vi "Fetch Multi Eval Meas List Segment SEM Margin Area Results.vi"(6 "Offset Frequency (Negative)":i32(ring) items=["Negative", "Positive"], 7 "Segment (1)":T2=1, 8 "error in (no error)":errorcluster, 9 "Result Type (Current)":i32(ring) items=["Current"=0, "Average"=1, "Minimum"=5], 10 "Instance (1)":T3=1, 11 "VISA resource name":refnum<visa-resource-name>) -> (0 "error out":errorcluster, 1 "SEM Offset Results":cluster{"Margin X":dbl, "Margin Y":dbl}[](array[cluster]) {"Margin Y" format="%^.3e"; "Margin X" format="%^.3e"}, 2 "Reliability Results":T1, 3 "VISA resource name out":refnum<visa-resource-name>, 4 "Statistic Expired":i32, 5 "Out Of Tolerance":dbl format="%^.3e")   [LabVIEW 2020, in "Rohde&Schwarz CMXP NR FR2 Measurement.lvlib"]
doc: "Returns spectrum emission mask margin results for segment <no> in list mode.\n\nAttributes:\nRSCMXPNRFR2M_ATTR_FETCH_MULTI_EVAL_MEASUREMENT_LIST_SEGMENT_SEM_NEGATIVE_CURRENT_RESULTS\nRSCMXPNRFR2M_ATTR_FETCH_MULTI_EVAL_MEASUREMENT_LIST_SEGMENT_SEM_NEGATIVE_AVERAGE_RESULTS\nRSCMXPNRFR2M_ATTR_FETCH_MULTI_EVAL_MEASUREMENT_LIST_SEGMENT_SEM_NEGATIVE_MINIMUM_RESULTS\nRSCMXPNRFR2M_ATTR_FETCH_MULTI_EVAL_MEASUREMENT_LIST_SEGMENT_SEM_POSITIVE_CURRENT_RESULTS\nRSCMXPNRFR2M_ATTR_FETCH_MULTI_EVAL_MEASUREMENT_LIST_SEGMENT_SEM_POSITIVE_AVERAGE_RESULTS\nRSCMXPNRFR2M_ATTR_FETCH_MULTI_EVAL_MEASUREMENT_LIST_SEGMENT_SEM_POSITIVE_MINIMUM_RESULTS\n\nRemote-control commands:\nFETCh:NRMMw:MEAS<i>:MEValuation:LIST:SEGMent<no>:SEMask:MARGin:CURRent:NEGativ?\nFETCh:NRMMw:MEAS<i>:MEValuation:LIST:SEGMent<no>:SEMask:MARGin:AVERage:NEGativ?\nFETCh:NRMMw:MEAS<i>:MEValuation:LIST:SEGMent<no>:SEMask:MARGin:MINimum:NEGativ?\nFETCh:NRMMw:MEAS<i>:MEValuation:LIST:SEGMent<no>:SEMask:MARGin:CURRent:POSitiv?\nFETCh:NRMMw:MEAS<i>:MEValuation:LIST:SEGMent<no>:SEMask:MARGin:AVERage:POSitiv?\nFETCh:NRMMw:MEAS<i>:MEValuation:LIST:SEGMent<no>:SEMask:MARGin:MINimum:POSitiv?"
uses:
  <instrlib>/Rohde&Schwarz CMXP NR FR2 Measurement/Rohde&Schwarz CMXP NR FR2 Measurement.lvlib
  <instrlib>/Rohde&Schwarz CMXP NR FR2 Measurement/Private/_Instance.ctl
  <instrlib>/Rohde&Schwarz CMXP NR FR2 Measurement/Private/_Segment.ctl
  <instrlib>/Rohde&Schwarz CMXP NR FR2 Measurement/Private/rsidr_core.llb/rsidr_core.lvlib
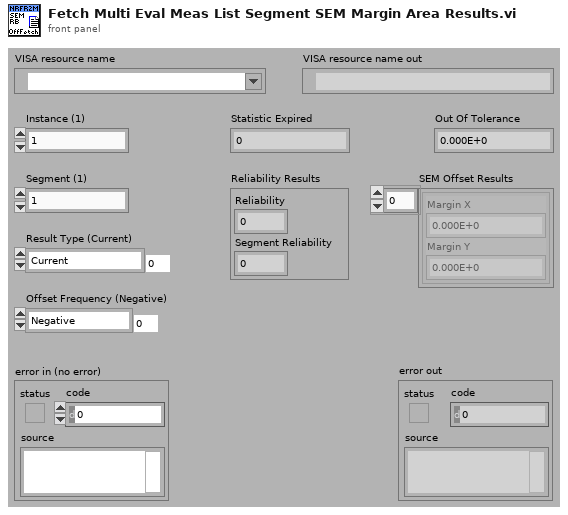
[diagram p1: front panel]
types:
  T1 = cluster{"Reliability":i32, "Segment Reliability":i32}
  T2 = typedef "Rohde&Schwarz CMXP NR FR2 Measurement.lvlib/_Segment.ctl" = i32
  T3 = typedef "Rohde&Schwarz CMXP NR FR2 Measurement.lvlib/_Instance.ctl" = i32
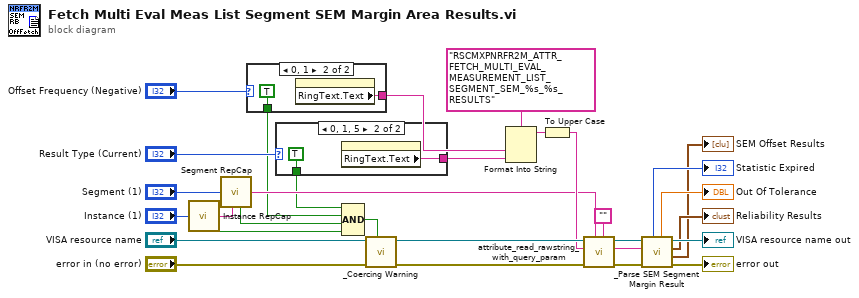
[diagram p0: block diagram]
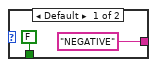
[diagram p2: hidden frame]
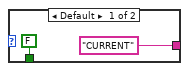
[diagram p3: hidden frame]
diagram:
  n1 = call <instrlib>:"Instance RepCap.vi"("Instance In"="Instance (1)") -> ("In Range?"=w24:bool, "RepCap Identifier Out"=w1:string)  [unwired: 1 in]
  n2 = call <instrlib>:"Segment RepCap.vi"("Segment In"="Segment (1)", "RepCap String In (\"\")"=w1) -> ("In Range?"=w23:bool, "RepCap Identifier Out"=w10:string)
  n3 = case shown="0, 1" "Offset Frequency (Negative)" {
    tunnel: ["NEGATIVE" w33] -> w5
    tunnel: [FALSE TRUE] -> w4
    frame Default {
    }
    frame 0, 1 {
      n4 = property on="Offset Frequency (Negative)" class="Ring (strict)"() -> ("RingText.Text"=w33:string)  [unwired: 2 in, 2 out]
    }
  }
  n5 = case shown="0, 1, 5" "Result Type (Current)" {
    tunnel: ["CURRENT" w37] -> w26
    tunnel: [FALSE TRUE] -> w3
    frame Default {
    }
    frame 0, 1, 5 {
      n6 = property on="Result Type (Current)" class="Ring (strict)"() -> ("RingText.Text"=w37:string)  [unwired: 2 in, 2 out]
    }
  }
  n7 = Compound Arithmetic op=AND(w3, w4, w23, w24) -> (w22:bool)
  n8 = call <instrlib>:"_Coercing Warning.vi"("In Range?"=w22, "error in (no error)"="error in (no error)", "VISA resource name"="VISA resource name") -> ("error out"=w18:errorcluster, "VISA resource name out"=w17:refnum<visa-resource-name>)  [unwired: 7 in]
  n9 = Format Into String(format string="RSCMXPNRFR2M_ATTR_FETCH_MULTI_EVAL_MEASUREMENT_LIST_SEGMENT_SEM_%s_%s_RESULTS", w5, w26) -> (resulting string=w25:string)  [unwired: 2 in, 1 out]
  n10 = To Upper Case(1:w25) -> (0:w16:string)
  n11 = call <instrlib>:"attribute_read_rawstring_with_query_param.vi"("Query Parameter (None)"="" ("Empty String Constant"), "Repeated Capability"=w10, "error in"=w18, "Attribute ID"=w16, "VISA resource name"=w17) -> ("error out"=w15:errorcluster, "Raw String out"=w14:string, "VISA resource name out"=w13:refnum<visa-resource-name>)  [unwired: 4 in]
  n12 = call <instrlib>:"_Parse SEM Segment Margin Result.vi"("error in (no error)"=w15, "Input String"=w14, "VISA resource name"=w13) -> ("error out"=→"error out":errorcluster, "SEM Offset Results"=→"SEM Offset Results":cluster{"Margin X":dbl, "Margin Y":dbl}[], "Reliability Results"=→"Reliability Results":T1, "VISA resource name out"=→"VISA resource name out":refnum<visa-resource-name>, "Out Of Tolerance"=→"Out Of Tolerance":dbl, "Statistic Expired"=→"Statistic Expired":i32)  [unwired: 3 in]
